vi "EnStringQueue.vi"(8 "error in":errorcluster, 9 "StringIn":string, 11 "QueueIn":variant) -> (0 "error out":errorcluster, 3 "QueueOut":variant)   [LabVIEW 2013]
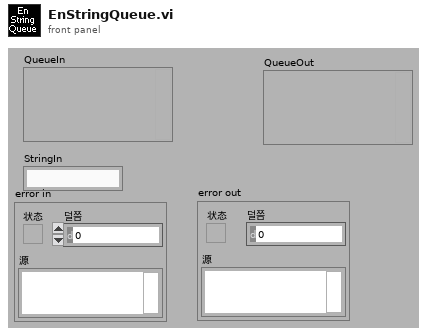
[diagram p1: front panel]
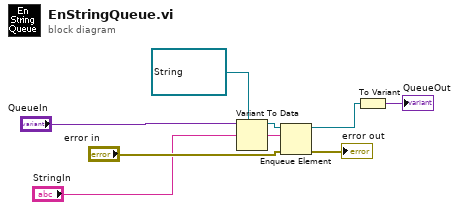
[diagram p0: block diagram]
diagram:
  n1 = Variant To Data(type=refnum<queue> refnum ("queue out"), Variant="QueueIn") -> (data=w1:refnum<queue>)  [unwired: 1 in, 1 out]
  n2 = Enqueue Element(queue=w1, element="StringIn", error in (no error)="error in") -> (queue out=w3:refnum<queue>, error out=→"error out":errorcluster)  [unwired: 2 out]
  n3 = To Variant(anything=w3) -> (Variant=→"QueueOut":variant)
